vi "test.SocketDebug.vi"() -> ()   [LabVIEW 2014]
uses:
  Private/Class/meth.Constructor.vi
  Private/Class/meth.ExecFromFile.vi
  Private/Class/meth.Destructor.vi
  GLue.lvlib
panel:
  out "Return Data":variant
  out "error out":errorcluster
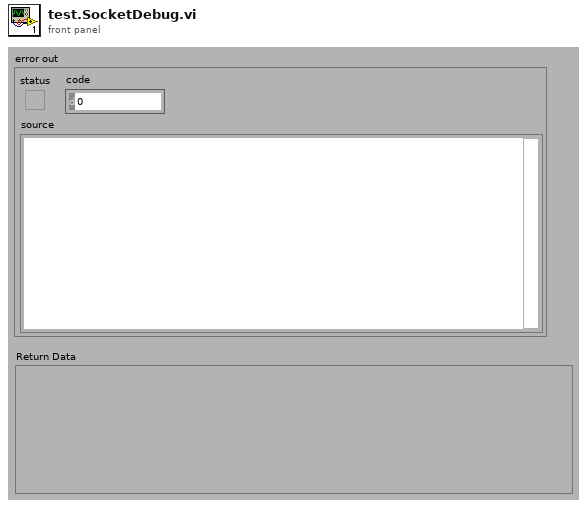
[diagram p1: front panel]
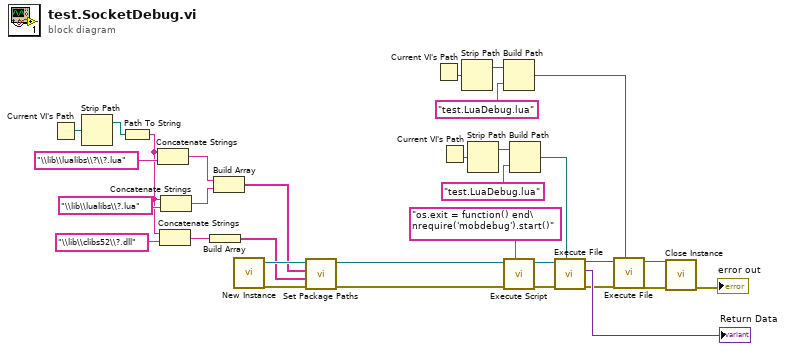
[diagram p0: block diagram]
diagram:
  n1 = Current VI's Path() -> (path=w31:path)
  n2 = Strip Path(path=w31) -> (stripped path=w29:path)  [unwired: 1 out]
  n3 = Path To String(path=w29) -> (string=w26:string)
  n4 = Concatenate Strings(w26, "\\lib\\lualibs\\?\\?.lua" ("string")) -> (w21:string)
  n5 = Concatenate Strings(w26, "\\lib\\clibs52\\?.dll" ("string")) -> (w22:string)
  n6 = Concatenate Strings(w26, "\\lib\\lualibs\\?.lua" ("string")) -> (w20:string)
  n7 = Build Array(w22) -> (w19:string[])
  n8 = Build Array(w21, w20) -> (w18:string[])
  n9 = call "New Instance.vi"() -> ("error out"=w23:errorcluster, "GLue out"=w24:refnum<class "class.GLue.lvclass">)  [unwired: 10 in]
  n10 = call "Set Package Paths.vi"("error in"=w23, "Cpaths"=w19, "Lpaths"=w18, "GLue in"=w24) -> ("error out"=w1:errorcluster, "GLue out"=w2:refnum<class "class.GLue.lvclass">)  [unwired: 6 in]
  n11 = Current VI's Path() -> (path=w4:path)
  n12 = Current VI's Path() -> (path=w17:path)
  n13 = Strip Path(path=w4) -> (stripped path=w5:path)  [unwired: 1 out]
  n14 = Strip Path(path=w17) -> (stripped path=w16:path)  [unwired: 1 out]
  n15 = Build Path(base path=w5, name or relative path="test.LuaDebug.lua") -> (appended path=w3:path)
  n16 = call "Execute Script.vi"("Script"="os.exit = function() end\nrequire('mobdebug').start()", "error in"=w1, "GLue in"=w2) -> ("error out"=w13:errorcluster, "GLue out"=w12:refnum<class "class.GLue.lvclass">)  [unwired: 6 in, 1 out]
  n17 = Build Path(base path=w16, name or relative path="test.LuaDebug.lua") -> (appended path=w15:path)
  n18 = call "Execute File.vi"("Path"=w15, "error in"=w13, "GLue in"=w12) -> ("error out"=w10:errorcluster, "Return Data"=→"Return Data":variant, "GLue out"=w9:refnum<class "class.GLue.lvclass">)  [unwired: 6 in]
  n19 = call "Execute File.vi"("Path"=w3, "error in"=w10, "GLue in"=w9) -> ("error out"=w7:errorcluster, "GLue out"=w8:refnum<class "class.GLue.lvclass">)  [unwired: 6 in, 1 out]
  n20 = call "Close Instance.vi"("error in"=w7, "GLue in"=w8) -> ("error out"=→"error out":errorcluster)  [unwired: 9 in]
